vi "Actor Core.vi"(8 "error in":errorcluster, 11 "About View in":refnum<class "About View.lvclass">) -> (0 "error out":errorcluster, 3 "Actor out":refnum<class "Actor.lvclass">)   [LabVIEW 2020, in "About View.lvlib" / "About View.lvclass"]
doc: "(<B>Filename</B>: Actor Framework.lvlib:Actor.lvclass:Actor Core.vi)\n\nReceives messages to the actor, reacts to them, and initiates any error handling that may shut the actor down.\n\nDescendant classes may override this VI to append parallel tasks for the actor to complete while it handles messages. Overrides use the Call Parent Method node."
uses:
  About View.lvclass
  C:/Program Files/National Instruments/LabVIEW 2020/vi.lib/ActorFramework/Actor/Actor.lvclass
  <vilib>/ActorFramework/Actor/Actor.lvclass
  About View.lvclass/About View.ctl
  <vilib>/ActorFramework/Actor/Actor.lvclass/Actor.ctl
  <vilib>/ActorFramework/Message Enqueuer/Message Enqueuer.lvclass/Message Enqueuer.ctl
  About View Messages/Broadcast Map Yaml Msg/Broadcast Map Yaml Msg.lvclass/Broadcast Map Yaml Msg.ctl
  <vilib>/ActorFramework/Message Enqueuer/Init from Existing Queue.vi
  <vilib>/ActorFramework/Message Enqueuer/Enqueue.vi
  About View Messages/Broadcast Map Yaml Msg/Broadcast Map Yaml Msg.lvclass
  C:/Program Files/National Instruments/LabVIEW 2020/vi.lib/ActorFramework/Message/Message.lvclass
  <vilib>/ActorFramework/Message Priority Queue/Priority Enqueue.vi
  <vilib>/ActorFrameworkMVC/Abstract View/Abstract View/Abstract View.lvclass
  <vilib>/ActorFramework/Message Enqueuer/Message Enqueuer.lvclass
panel:
  in  "Map Yaml":T1
  in  "Update Button":bool
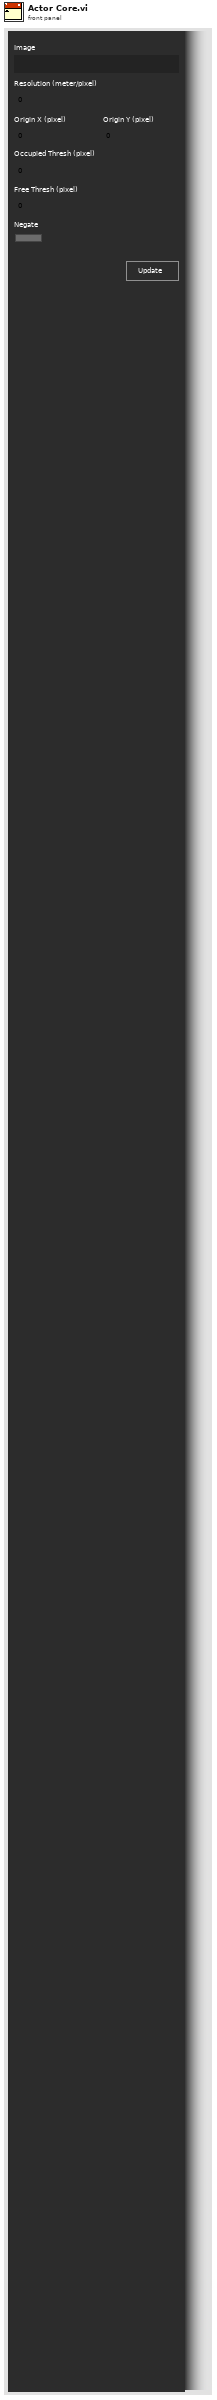
[diagram p1: front panel]
types:
  T1 = cluster{"Image":string, "Resolution (meter/pixel)":dbl, "Origin":cluster{"Origin X (pixel)":dbl, "Origin Y (pixel)":dbl, "Origin R":dbl}, "Occupied Thresh (pixel)":dbl, "Free Thresh (pixel)":dbl, "Negate":bool}
  T2 = enum8{"Enabled", "Disabled", "Disabled and Grayed Out"}
  T3 = cluster{"Map Yaml":cluster{"Image":string, "Resolution (meter/pixel)":dbl, "Origin":cluster{"Origin X (pixel)":dbl, "Origin Y (pixel)":dbl, "Origin R":dbl}, "Occupied Thresh (pixel)":dbl, "Free Thresh (pixel)":dbl, "Negate":bool}}
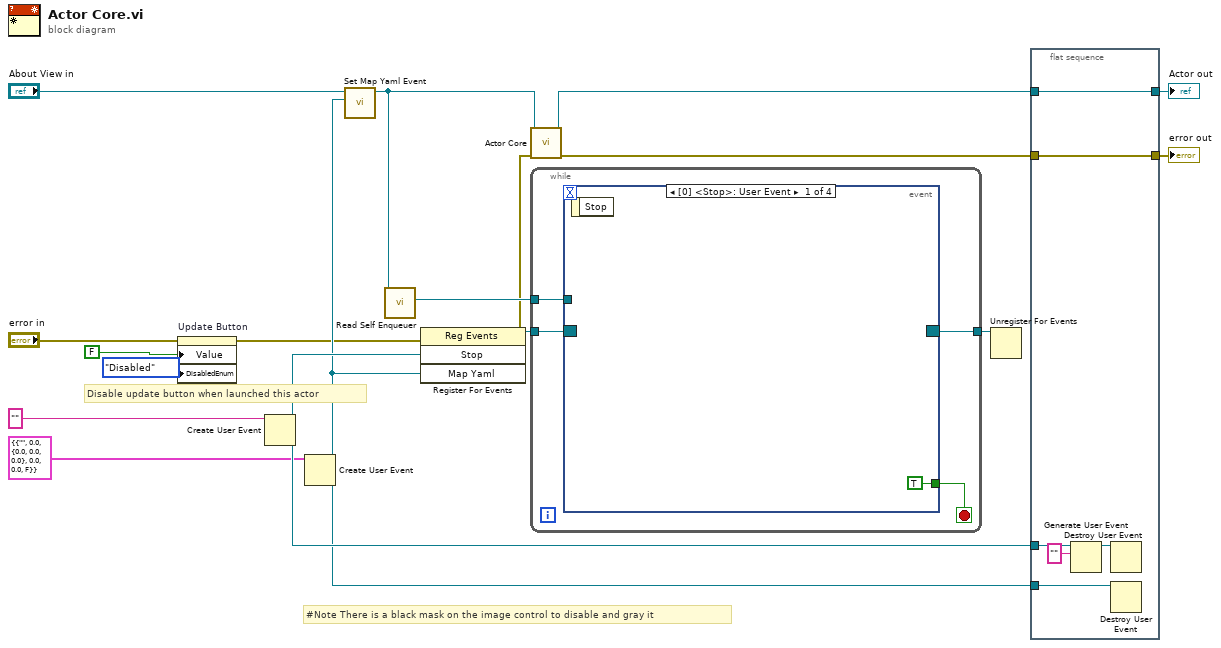
[diagram p0: block diagram]
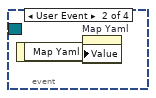
[diagram p2: hidden frame]
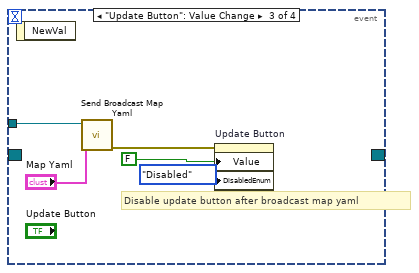
[diagram p3: hidden frame]
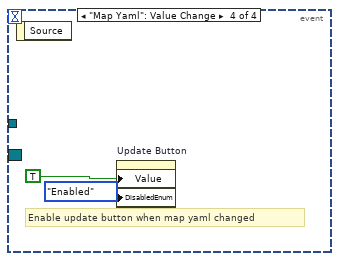
[diagram p4: hidden frame]
diagram:
  # "#Note There is a black mask on the image control to disable and gray it"
  # "Disable update button when launched this actor"
  n1 = property on="Update Button" class="Bool (strict)"(error in="error in", "Value"=FALSE ("Update Button"), "DisabledEnum"=T2."Disabled" ("Disabled")) -> (error out=w1:errorcluster)  [unwired: 1 in, 1 out]
  n2 = Create User Event(user event datatype="" ("Stop")) -> (user event=w12:refnum<user-event>)  [unwired: 1 in, 1 out]
  n3 = Create User Event(user event datatype=T3 {"Map Yaml"={"Image"="", "Resolution (meter/pixel)"=0.0, "Origin"={"Origin X (pixel)"=0.0, "Origin Y (pixel)"=0.0, "Origin R"=0.0}, "Occupied Thresh (pixel)"=0.0, "Free Thresh (pixel)"=0.0, "Negate"=FALSE}} ("Map Yaml")) -> (user event=w5:refnum<user-event>)  [unwired: 1 in, 1 out]
  n4 = call "Set Map Yaml Event.vi"("Map Yaml Event"=w5, "About View in"="About View in") -> ("About View out"=w9:refnum<class "About View.lvclass">)  [unwired: 9 in]
  n5 = call <vilib>:"Read Self Enqueuer.vi"("Actor"=w9) -> ("Self Enqueuer"=w13:refnum<class "Message Enqueuer.lvclass">)  [unwired: 10 in]
  n6 = register-events(error in=w1, w12, w5) -> (reference out=w16:refnum<event-registration>, error out=w11:errorcluster)  [unwired: 1 in]
  n7 = call-parent "Actor Core.vi"("error in"=w11, "Abstract View in"=w9) -> ("error out"=w14:errorcluster, "Actor out"=w15:refnum<class "Actor.lvclass">)  [unwired: 8 in]
  n8 = while {
    tunnel: w16 -> [w22]
    tunnel: [w21] -> w17
    tunnel: w13 -> [w19]
    stop <- w20 stop-if-true
    n9 = event shown="[0] <Stop>: User Event" {
      selector: w22 -> [_ _ _ _]
      dyn-events: [_ _ _ _] -> w21
      timeout: _ -> [_ _ _ _]
      tunnel: [TRUE _ _ _] -> w20
      tunnel: w19 -> [_ _ w29 _]
      event User Event {
        n10 = event-data() -> ()  [unwired: 1 in, 1 out]
      }
      event User Event {
        n11 = event-data() -> ("Map Yaml"=w24:T1)  [unwired: 1 in]
        n12 = property on="Map Yaml" class="Clust (strict)"("Value"=w24) -> ()  [unwired: 2 in, 2 out]
      }
      event "Update Button": Value Change {
        # "Disable update button after broadcast map yaml"
        n13 = event-data() -> ()  [unwired: 1 in, 1 out]
        n14 = call "Send Broadcast Map Yaml.vi"("Map Yaml"="Map Yaml", "Message Enqueuer"=w29) -> ("error out"=w25:errorcluster)  [unwired: 8 in, 1 out]
        n15 = property on="Update Button" class="Bool (strict)"(error in=w25, "Value"=FALSE ("Update Button"), "DisabledEnum"=T2."Disabled" ("Disabled")) -> ()  [unwired: 1 in, 2 out]
      }
      event "Map Yaml": Value Change {
        # "Enable update button when map yaml changed"
        n16 = event-data() -> ()  [unwired: 1 in, 1 out]
        n17 = property on="Update Button" class="Bool (strict)"("Value"=TRUE ("Update Button"), "DisabledEnum"=T2."Enabled" ("Disabled")) -> ()  [unwired: 2 in, 2 out]
      }
    }
  }
  n18 = Unregister For Events(event registration refnum=w17) -> ()  [unwired: 1 in, 1 out]
  n19 = flat-sequence {
    tunnel: w12 -> [w36]
    tunnel: w5 -> [w34]
    tunnel: w15 -> [w33]
    tunnel: [w33] -> w8
    tunnel: [w32] -> w7
    tunnel: w14 -> [w32]
    frame #0 {
      n20 = Generate User Event(user event=w36, event data cluster="" ("event data")) -> (user event out=w37:refnum<user-event>)  [unwired: 2 in, 1 out]
      n21 = Destroy User Event(user event=w37) -> ()  [unwired: 1 in, 1 out]
      n22 = Destroy User Event(user event=w34) -> ()  [unwired: 1 in, 1 out]
    }
  }
  "error out" <- w7
  "Actor out" <- w8
